vi "svfa_Check Data Valid [Dual Zoom].vi"(0 "stimulus [X]":waveform(dbl)={"t0"=timestamp(0 s since 1904-01-01), "dt"=1.953125e-05, "Y"=[]}, 1 "response [Y]":waveform(dbl)={"t0"=timestamp(0 s since 1904-01-01), "dt"=1.953125e-05, "Y"=[]}, 2 "measurement":T1(ring)=enum."Frequency response", 4 "averaging parameters":T2={"averaging mode"=enum."No averaging", "weighting mode"=enum."Linear", "number of averages"=10, "linear mode"=enum."Auto restart"}, 5 "error in (no error)":errorcluster, 6 "restart averaging (F)":bool, 7 "zoom settings":T4={"frequency range"={"start frequency"=1000.0, "stop frequency"=2000.0}, "window"=1, "number of lines"=400, "% overlap"=0.0} {"% overlap" min=0.0 format="%.2f"; "number of lines" min=2; "window" items=["None ", "Hanning", "Hamming", "Blackman-Harris", "Exact Blackman", "Blackman", "Flat Top", "4 Term B-Harris ", "7 Term B-Harris", "Low Sidelobe"]; "frequency range"."stop frequency" min=0.0 format="%.2f"; "frequency range"."start frequency" min=0.0 format="%.2f"}, 9 "FRF mode":enum16{"H1", "H2", "H3"}(ring)) -> (10 "reset processing":bool, 11 "dup FRF mode":enum16{"H1", "H2", "H3"}(ring), 12 "restart averaging":bool, 13 "zoom FFT settings":T3={"zoom settings"={"center frequency"=-inf, "zoom"=1, "trim"=1.0}, "FFT settings"={"window"=enum."Hanning", "window size"=-1, "FFT size"=1024, "%overlap"=0.0}} {"FFT settings"."%overlap" min=0.0 max=100.0 format="%.2f"; "zoom settings"."trim" min=1.0 format="%.2f"; "zoom settings"."center frequency" format="%.2f"; "zoom settings"."zoom" min=1}, 14 "dup stimulus [X]":waveform(dbl)={"t0"=timestamp(0 s since 1904-01-01), "dt"=1.953125e-05, "Y"=[]}, 15 "dup response [Y]":waveform(dbl)={"t0"=timestamp(0 s since 1904-01-01), "dt"=1.953125e-05, "Y"=[]}, 16 "iterations":i32, 17 "maximum block size":i32, 18 "dup averaging parameters":T2={"averaging mode"=enum."No averaging", "weighting mode"=enum."Linear", "number of averages"=10, "linear mode"=enum."Auto restart"}, 19 "error out":errorcluster)   [LabVIEW 2017]
uses:
  <vilib>/addons/_NISVFA/_Shared subVIs/Common/svc_Check for Waveform Parameter Continuity (1 Ch).vi
  <vilib>/addons/_NISVFA/_Shared subVIs/Common/svc_Check for Waveform Parameter Continuity (no state).vi
  <vilib>/addons/_NISVFA/_Shared subVIs/Common/svc_Get SV Channel Info.vi
  <vilib>/addons/_NISVFA/_Shared subVIs/Common/svc_Check dt for Equal Sample Rates.vi
  <vilib>/addons/_NISVFA/_Shared subVIs/Common/svc_Engineering Units to Unit Label.vi
  <vilib>/addons/_NISVFA/_Shared subVIs/Common/svc_Unit Label to Engineering Units.vi
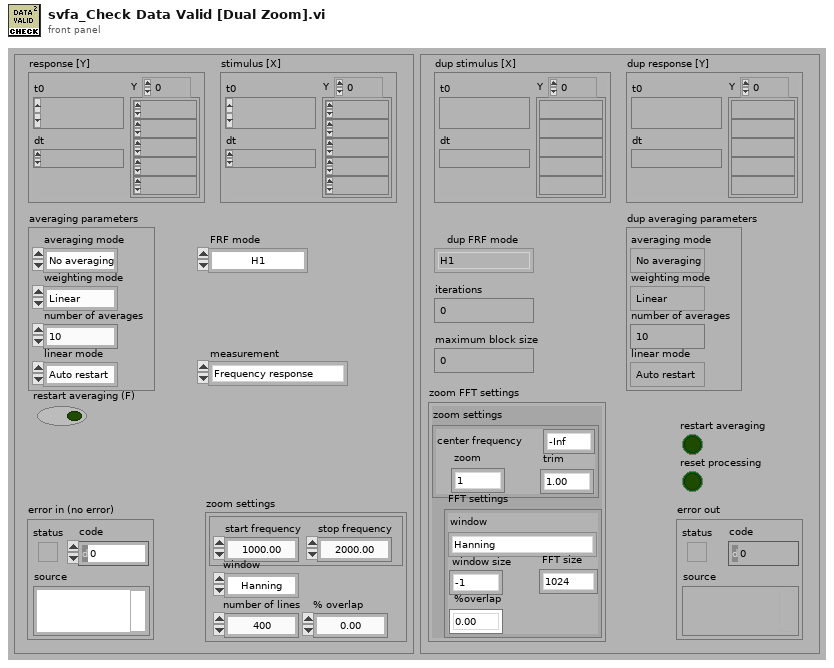
[diagram p1: front panel]
types:
  T1 = enum16{"Cross spectrum", "Frequency response", "Coherent output power"}
  T2 = cluster{"averaging mode":enum16{"No averaging", "Vector averaging", "RMS averaging", "Peak hold"}, "weighting mode":enum16{"Linear", "Exponential"}, "number of averages":u32, "linear mode":enum16{"One shot", "Auto restart"}}
  T3 = cluster{"zoom settings":cluster{"center frequency":dbl, "zoom":i32, "trim":dbl}, "FFT settings":cluster{"window":enum16{"None ", "Hanning", "Hamming", "Blackman-Harris", "Exact Blackman", "Blackman", "Flat Top", "4 Term B-Harris ", "7 Term B-Harris", "Low Sidelobe"}, "window size":i32, "FFT size":i32, "%overlap":dbl}}
  T4 = cluster{"frequency range":cluster{"start frequency":dbl, "stop frequency":dbl}, "window":u16, "number of lines":i32, "% overlap":dbl}
  T5 = cluster{"dt":bool, "t0 continuity":bool, "array length":bool, "channel info":bool, "name":bool}
  T6 = typedef "NI_AALPro.lvlib/windowTd.ctl" = u32
  T7 = enum16{"No averaging", "Vector averaging", "RMS averaging", "Peak hold"}
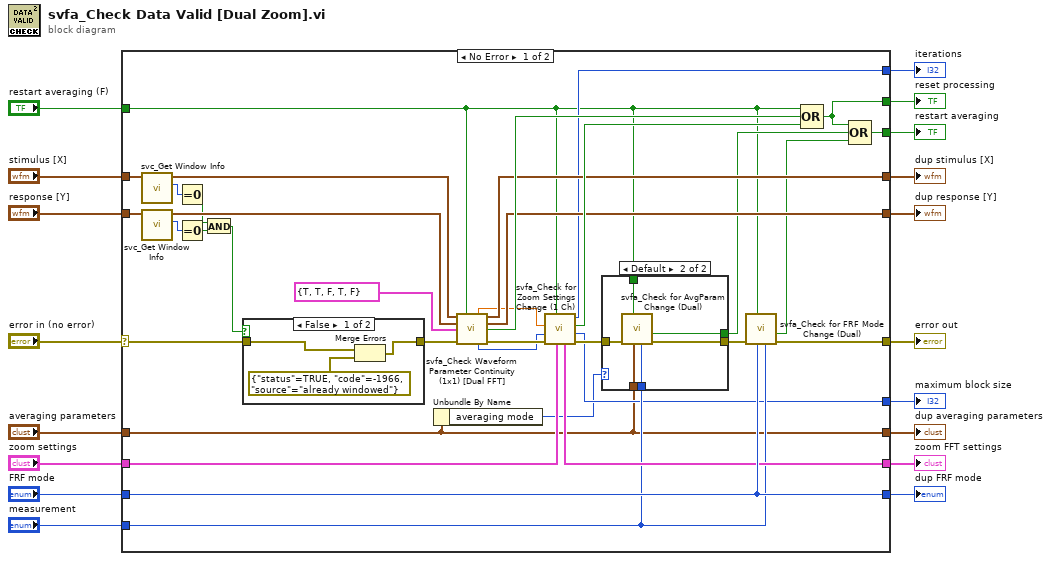
[diagram p0: block diagram]
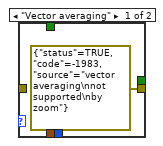
[diagram p2: hidden frame]
diagram:
  n1 = case shown="No Error" "error in (no error)" {
    selector: "error in (no error)" -> [w31 w70]
    tunnel: [w20 w70] -> w11
    tunnel: "stimulus [X]" -> [w37 w67]
    tunnel: "response [Y]" -> [w39 w66]
    tunnel: "restart averaging (F)" -> [w19 w65]
    tunnel: "zoom settings" -> [w52 _]
    tunnel: [w51 _] -> w12
    tunnel: [w53 w69] -> w10
    tunnel: "FRF mode" -> [w53 w69]
    tunnel: "averaging parameters" -> [w22 w68]
    tunnel: [w22 w68] -> w9
    tunnel: "measurement" -> [w50 _]
    tunnel: [w42 w67] -> w7
    tunnel: [w43 w66] -> w5
    tunnel: [w26 _] -> w4
    tunnel: [w25 _] -> w3
    tunnel: [w24 w65] -> w2
    tunnel: [w23 w65] -> w1
    frame No Error {
      n2 = call <vilib>:"svc_Get Window Info.vi"("scaled signal [EU]"=w37) -> ("window"=w33:T6, "dup scaled signal [EU]"=w36:waveform(dbl))  [unwired: 6 in, 3 out]
      n3 = call <vilib>:"svc_Get Window Info.vi"("scaled signal [EU]"=w39) -> ("window"=w35:T6, "dup scaled signal [EU]"=w38:waveform(dbl))  [unwired: 6 in, 3 out]
      n4 = Equal To 0?(x=w33) -> (x = 0?=w30:bool)
      n5 = Equal To 0?(x=w35) -> (x = 0?=w34:bool)
      n6 = And(x=w30, y=w34) -> (x .and. y?=w32:bool)
      n7 = case shown="False" w32 {
        tunnel: w31 -> [w62 w64]
        tunnel: [w63 w64] -> w29
        frame False {
          n8 = Merge Errors(w62, errorcluster {"status"=TRUE, "code"=-1966, "source"="already windowed"} ("error in 2 (no error)")) -> (w63:errorcluster)
        }
        frame True {
        }
      }
      n9 = Unbundle By Name(w22) -> ("averaging mode"=w21:T7)
      n10 = call <vilib>:"svfa_Check Waveform Parameter Continuity (1x1) [Dual FFT].vi"("stimulus signal X [EUx]"=w36, "restart averaging (F)"=w19, "response signal Y [EUy]"=w38, "checks for channel parameter change"=T5 {"dt"=TRUE, "t0 continuity"=TRUE, "array length"=FALSE, "channel info"=TRUE, "name"=FALSE}, "error in"=w29) -> ("dt"=w41:dbl, "stimulus signal X [EUx]"=w42:waveform(dbl), "response signal Y [EUy]"=w43:waveform(dbl), "waveform parameter changed"=w44:bool, "array length"=w40:i32, "error out"=w46:errorcluster)  [unwired: 5 in]
      n11 = call <vilib>:"svfa_Check for Zoom Settings Change (1 Ch).vi"("zoom settings"=w52, "restart averaging (F)"=w19, "error in (no error)"=w46, "array length"=w40, "dt"=w41) -> ("error out"=w49:errorcluster, "maximum block size"=w26:i32, "zoom settings changed"=w45:bool, "iterations"=w25:i32, "zoom FFT settings"=w51:T3)  [unwired: 2 in]
      n12 = case shown="Default" w21 {
        tunnel: w50 -> [_ w60]
        tunnel: w49 -> [_ w59]
        tunnel: [errorcluster {"status"=TRUE, "code"=-1983, "source"="vector averaging\nnot supported\nby zoom"} ("error IO") w58] -> w48
        tunnel: [_ w57] -> w28
        tunnel: w19 -> [_ w56]
        tunnel: w22 -> [_ w55]
        frame "Vector averaging" {
        }
        frame Default {
          n13 = call <vilib>:"svfa_Check for AvgParam Change (Dual).vi"("measurement"=w60, "averaging parameters"=w55, "restart averaging (F)"=w56, "error in (no error)"=w59) -> ("error out"=w58:errorcluster, "parameter has changed"=w57:bool)  [unwired: 6 in]
        }
      }
      n14 = call <vilib>:"svfa_Check for FRF Mode Change (Dual).vi"("measurement"=w50, "FRF mode"=w53, "restart"=w19, "error in (no error)"=w48) -> ("error out"=w20:errorcluster, "parameter has changed"=w27:bool)  [unwired: 6 in]
      n15 = Compound Arithmetic op=OR(w19, w44, w45) -> (w24:bool)
      n16 = Compound Arithmetic op=OR(w24, w28, w27) -> (w23:bool)
    }
    frame Error {
    }
  }
  "dup stimulus [X]" <- w7
  "error out" <- w11
  "dup response [Y]" <- w5
  "dup averaging parameters" <- w9
  "zoom FFT settings" <- w12
  "dup FRF mode" <- w10
  "iterations" <- w3
  "maximum block size" <- w4
  "reset processing" <- w2
  "restart averaging" <- w1
